vi "BNO055 Init.vi"(7 "I2C Channel":u8=1, 8 "error in (no error)":errorcluster, 9 "BNO055 Config Options":T1={"I2C"={"Slave Address"=72, "Channel"=1}, "ADC"={"Channel"=4, "Expected Range (Programmable Gain Amplifier)"=0, "Sampling Mode"=1, "Sampling Rate"=4, "Comparator Mode"=1, "Comparator Polarity"=1, "Latching Comparator"=1, "Comparator Queue & Disable"=3}} {"ADC"."Comparator Queue & Disable" items=["Assert after one conversion", "Assert after two conversions", "Assert after four conversions", "Comparator disabled"]; "ADC"."Latching Comparator" items=["Non-latching", "Latching"]; "ADC"."Comparator Polarity" items=["Active Low", "Active High"]; "ADC"."Comparator Mode" items=["Traditional Comparator w/ hysteresis", "Window Comparator"]; "ADC"."Sampling Rate" items=["128SPS", "250SPS", "490SPS", "920SPS", "1600SPS", "2400SPS", "3300SPS"]; "ADC"."Sampling Mode" items=["Continuous Conversion", "Single-shot (Low Power)"]; "ADC"."Expected Range (Programmable Gain Amplifier)" items=["+/-6.144V", "+/-4.096V", "+/-2.048V", "+/-1.024V", "+/-0.512V", "+/-0.256V"]; "ADC"."Channel" items=["Differential: Ch 0&1", "Differential: Ch 0&3", "Differential: Ch 1&3", "Differential: Ch 2&3", "Single Ended: Ch 0", "Single Ended: Ch 1", "Single Ended: Ch 2", "Single Ended: Ch 3"]; "I2C"."Slave Address" format="%.0x"}, 10 "I2C Slave Address":u8=40 format="%.0x", 11 "LINX Resource in":T2) -> (0 "error out":errorcluster, 1 "BNO055 Config Options 2":T1={"I2C"={"Slave Address"=72, "Channel"=1}, "ADC"={"Channel"=4, "Expected Range (Programmable Gain Amplifier)"=0, "Sampling Mode"=1, "Sampling Rate"=4, "Comparator Mode"=1, "Comparator Polarity"=1, "Latching Comparator"=1, "Comparator Queue & Disable"=3}} {"ADC"."Comparator Queue & Disable" items=["Assert after one conversion", "Assert after two conversions", "Assert after four conversions", "Comparator disabled"]; "ADC"."Latching Comparator" items=["Non-latching", "Latching"]; "ADC"."Comparator Polarity" items=["Active Low", "Active High"]; "ADC"."Comparator Mode" items=["Traditional Comparator w/ hysteresis", "Window Comparator"]; "ADC"."Sampling Rate" items=["128SPS", "250SPS", "490SPS", "920SPS", "1600SPS", "2400SPS", "3300SPS"]; "ADC"."Sampling Mode" items=["Continuous Conversion", "Single-shot (Low Power)"]; "ADC"."Expected Range (Programmable Gain Amplifier)" items=["+/-6.144V", "+/-4.096V", "+/-2.048V", "+/-1.024V", "+/-0.512V", "+/-0.256V"]; "ADC"."Channel" items=["Differential: Ch 0&1", "Differential: Ch 0&3", "Differential: Ch 1&3", "Differential: Ch 2&3", "Single Ended: Ch 0", "Single Ended: Ch 1", "Single Ended: Ch 2", "Single Ended: Ch 3"]; "I2C"."Slave Address" format="%.0x"}, 3 "LINX Resource out":T2)   [LabVIEW 2014]
uses:
  <vilib>/MakerHub/LINX/Private/Type Defs/LINX Ref.ctl
  <vilib>/MakerHub/LINX/Private/Type Defs/Platform.ctl
  <vilib>/MakerHub/LINX/Private/Type Defs/Interface.ctl
  <vilib>/MakerHub/LINX/Private/Device/Type Defs/LINX Device Config.ctl
  <vilib>/MakerHub/LINX/Private/Device/Type Defs/TCP Config.ctl
  <vilib>/MakerHub/LINX/Private/Device/Type Defs/Channels.ctl
  BNO055 Config Options.ctl
  <vilib>/MakerHub/LINX/LMH-LINX.lvlib
  <vilib>/MakerHub/LINX/Private/Device/Device.lvlib
panel:
  # "NOT DONE\nYET!"
  # "NOT DONE\nYET!"
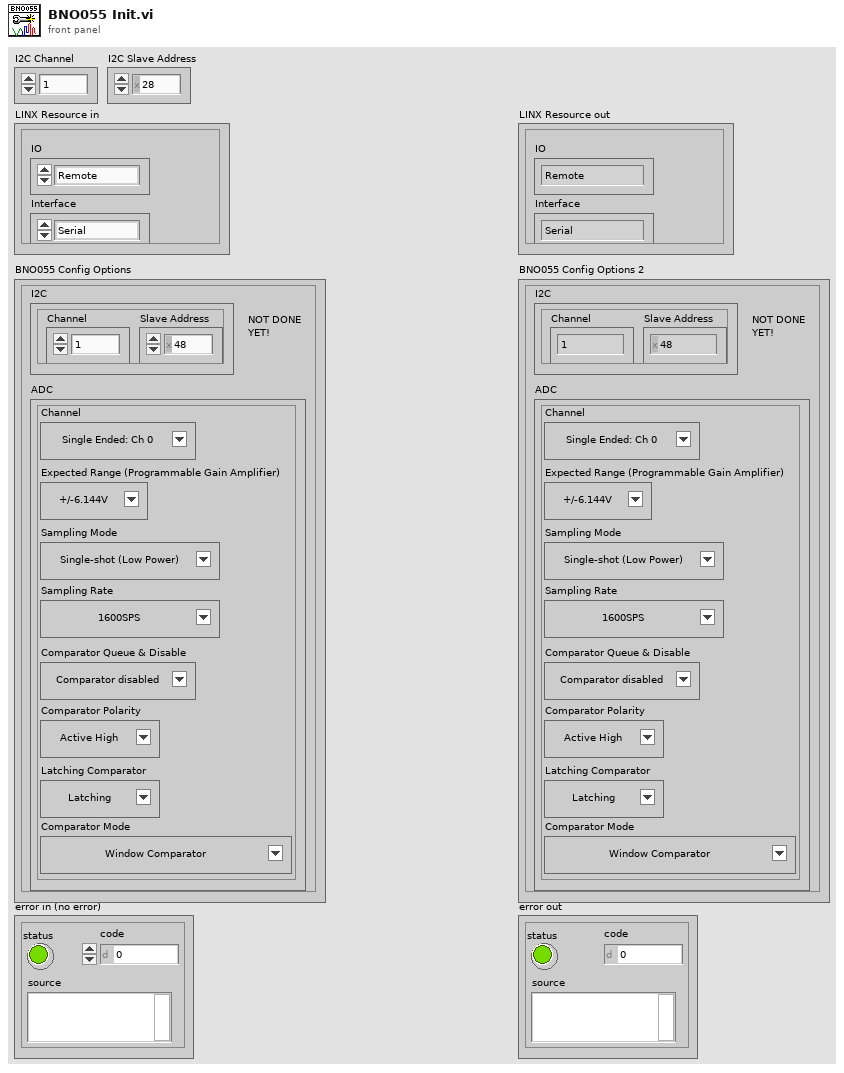
[diagram p1: front panel]
types:
  T1 = typedef "BNO055 Config Options.ctl" = cluster{"I2C":cluster{"Slave Address":u8, "Channel":u8}, "ADC":cluster{"Channel":u8, "Expected Range (Programmable Gain Amplifier)":u8, "Sampling Mode":u8, "Sampling Rate":u8, "Comparator Mode":u8, "Comparator Polarity":u8, "Latching Comparator":u8, "Comparator Queue & Disable":u8}}
  T2 = typedef "LMH-LINX.lvlib/LINX Ref.ctl" = cluster{"IO":T3, "Interface":T4, "LINX Device Config":T5}
  T3 = typedef "LMH-LINX.lvlib/Platform.ctl" = enum16{"Remote", "Local"}
  T4 = typedef "LMH-LINX.lvlib/Interface.ctl" = enum16{"Serial", "TCP"}
  T5 = typedef "LMH-LINX.lvlib/Device.lvlib/LINX Device Config.ctl" = cluster{"Interface":T4, "COM Port":refnum<visa-resource-name>, "TCP Configuration":T6, "Device Family":u8, "Device ID":u8, "Device Name":string, "TCP Ref":refnum<k5>, "Channels":T7}
  T6 = typedef "LMH-LINX.lvlib/Device.lvlib/TCP Config.ctl" = cluster{"IP Address":string, "Port":u16}
  T7 = typedef "LMH-LINX.lvlib/Channels.ctl" = cluster{"DI":u8[], "DO":u8[], "AI":u8[], "AO":u8[], "PWM":u8[], "QE":u8[], "UART":u8[], "I2C 2":u8[], "SPI":u8[], "CAN":u8[], "Servo":u8[], "AI Ref (V)":dbl, "AI Resolution (Bits)":u8, "AO Ref (V)":dbl, "AO Resolution (Bits)":u8}
  T8 = enum8{"Config", "Acc Only", "Mag Only", "Gyr Only", "AccMag", "AccGyr", "MagGyr", "AMG", "ImuPlus", "Compass", "M4G", "Ndof FMC Off", "NDOF"}
  T9 = enum8{"Config", "Acc Only", "Mag Only", "Gyr Only", "AccMag", "AccGyr", "MagGyr", "AMG", "ImuPlus", "Compass", "M4G", "Ndof FMC Off", "NDOF"}[]
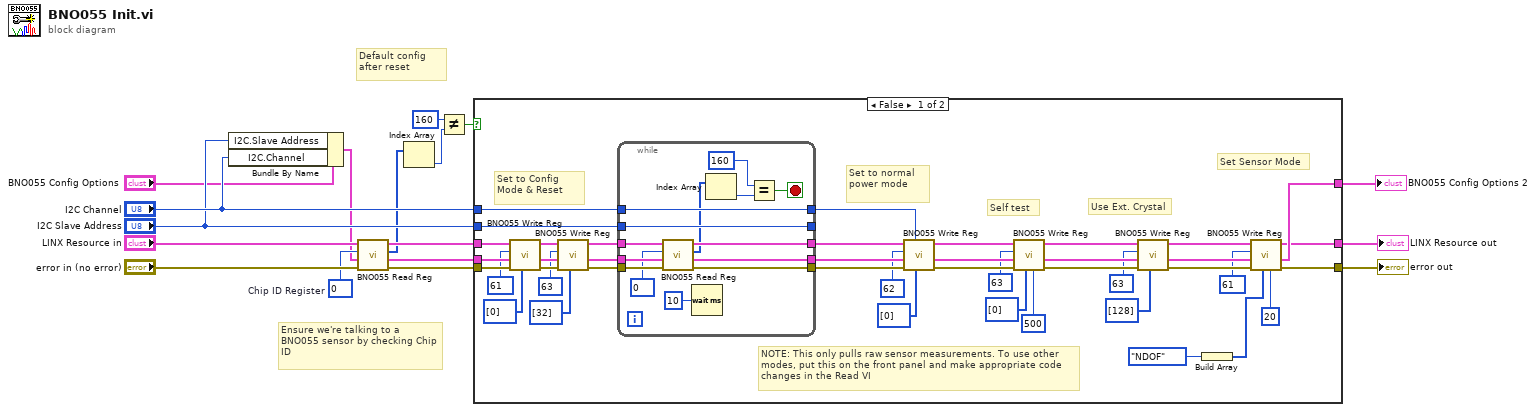
[diagram p0: block diagram]
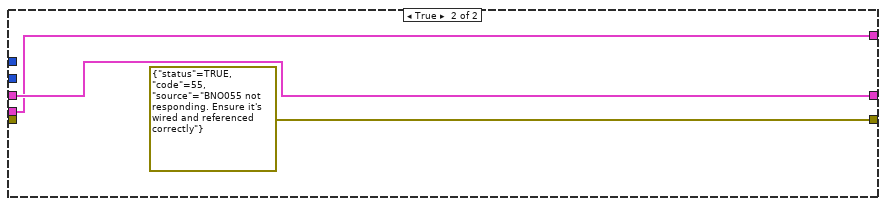
[diagram p2: hidden frame]
diagram:
  w8 = u8 0  # Chip ID Register
  # "Default config after reset"
  # "Ensure we're talking to a BNO055 sensor by checking Chip ID"
  n1 = Bundle By Name(cluster="BNO055 Config Options", "I2C.Slave Address"="I2C Slave Address", "I2C.Channel"="I2C Channel") -> (w7:T1)
  n2 = call "BNO055 Read Reg.vi"("error in (no error)"="error in (no error)", "BNO055 Config Options"=w7, "Register"=w8, "LINX Resource in"="LINX Resource in") -> ("error out"=w16:errorcluster, "BNO055 Config Options"=w3:T1, "Data out"=w5:u8[], "LINX Resource"=w6:T2)  [unwired: 4 in]
  n3 = Index Array(array=w5) -> (element=w4:u8)  [unwired: 1 in]
  n4 = Not Equal?(x=u8 160, y=w4) -> (x != y?=w15:bool)
  n5 = case shown="False" w15 {
    tunnel: w16 -> [w54 _]
    tunnel: [w45 errorcluster {"status"=TRUE, "code"=55, "source"="BNO055 not responding. Ensure it's wired and referenced correctly"} ("error constant")] -> w17
    tunnel: "I2C Channel" -> [w56 _]
    tunnel: "I2C Slave Address" -> [w57 _]
    tunnel: w6 -> [w53 w75]
    tunnel: w3 -> [w52 w74]
    tunnel: [w46 w74] -> w2
    tunnel: [w23 w75] -> w1
    frame False {
      # "Use Ext. Crystal"
      # "NOTE: This only pulls raw sensor measurements. To use other modes, put this on the front panel and make appropriate code changes in the Read VI"
      # "Set Sensor Mode"
      # "Self test"
      # "Set to normal power mode"
      # "Set to Config Mode & Reset"
      n6 = call "BNO055 Write Reg.vi"("Data"=u8[] [0], "error in (no error)"=w54, "BNO055 Config Options"=w52, "Register"=u8 61 ("I2C Slave Address 2"), "LINX Resource in"=w53) -> ("error out"=w40:errorcluster, "BNO055 Config Options"=w51:T1, "LINX Resource out"=w39:T2)  [unwired: 4 in]
      n7 = call "BNO055 Write Reg.vi"("Data"=u8[] [32], "error in (no error)"=w40, "BNO055 Config Options"=w51, "Register"=u8 63 ("I2C Slave Address 2"), "LINX Resource in"=w39) -> ("error out"=w41:errorcluster, "BNO055 Config Options"=w50:T1, "LINX Resource out"=w38:T2)  [unwired: 4 in]
      n8 = while {
        tunnel: w57 -> [w71]
        tunnel: w56 -> [w70]
        tunnel: [w71] -> _
        tunnel: [w70] -> w55
        tunnel: w50 -> [w68]
        tunnel: [w67] -> w49
        tunnel: [w66] -> w42
        tunnel: w41 -> [w65]
        tunnel: w38 -> [w64]
        tunnel: [w63] -> w37
        stop <- w69 stop-if-true
        n9 = call "BNO055 Read Reg.vi"("error in (no error)"=w65, "BNO055 Config Options"=w68, "Register"=u8 0 ("I2C Slave Address 2"), "LINX Resource in"=w64) -> ("error out"=w66:errorcluster, "BNO055 Config Options"=w67:T1, "Data out"=w61:u8[], "LINX Resource"=w63:T2)  [unwired: 4 in]
        n10 = Wait (ms)(milliseconds to wait=u32 10) -> ()  [unwired: 1 out]
        n11 = Index Array(array=w61) -> (element=w60:u8)  [unwired: 1 in]
        n12 = Equal?(x=u8 160, y=w60) -> (x = y?=w69:bool)
      }
      n13 = call "BNO055 Write Reg.vi"("Data"=u8[] [0], "Page"=w55, "error in (no error)"=w42, "BNO055 Config Options"=w49, "Register"=u8 62 ("I2C Slave Address 2"), "LINX Resource in"=w37) -> ("error out"=w31:errorcluster, "BNO055 Config Options"=w32:T1, "LINX Resource out"=w33:T2)  [unwired: 3 in]
      n14 = call "BNO055 Write Reg.vi"("Wait"=u32 500 ("milliseconds to wait"), "Data"=u8[] [0], "error in (no error)"=w31, "BNO055 Config Options"=w32, "Register"=u8 63 ("I2C Slave Address 2"), "LINX Resource in"=w33) -> ("error out"=w43:errorcluster, "BNO055 Config Options"=w48:T1, "LINX Resource out"=w36:T2)  [unwired: 3 in]
      n15 = call "BNO055 Write Reg.vi"("Data"=u8[] [128], "error in (no error)"=w43, "BNO055 Config Options"=w48, "Register"=u8 63 ("I2C Slave Address 2"), "LINX Resource in"=w36) -> ("error out"=w44:errorcluster, "BNO055 Config Options"=w47:T1, "LINX Resource out"=w35:T2)  [unwired: 4 in]
      n16 = Build Array(T8."NDOF") -> (w24:T9)
      n17 = call "BNO055 Write Reg.vi"("Wait"=u32 20, "Data"=w24, "error in (no error)"=w44, "BNO055 Config Options"=w47, "Register"=u8 61 ("I2C Slave Address 2"), "LINX Resource in"=w35) -> ("error out"=w45:errorcluster, "BNO055 Config Options"=w46:T1, "LINX Resource out"=w23:T2)  [unwired: 3 in]
    }
    frame True {
    }
  }
  "error out" <- w17
  "LINX Resource out" <- w1
  "BNO055 Config Options 2" <- w2
